vi "Write drive.vi"(8 "error in":errorcluster, 10 "drive":bool, 11 "PAS Data in":refnum<class "PAS Data.lvclass">) -> (0 "error out":errorcluster, 3 "PAS Data out":refnum<class "PAS Data.lvclass">)   [LabVIEW 2017, in "PAS Library.lvlib" / "PAS Data.lvclass"]
doc: "Write the current switch position (speaker or laser) to the data class for the PAS."
uses:
  PAS Data.lvclass
  PAS Data.lvclass/PAS Data.ctl
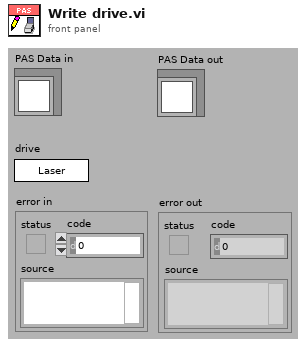
[diagram p1: front panel]
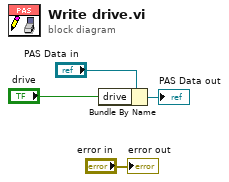
[diagram p0: block diagram]
diagram:
  n1 = Bundle By Name(cluster="PAS Data in", "drive"="drive") -> (→"PAS Data out":refnum<class "PAS Data.lvclass">)
  "error out" <- "error in"
